vi "PrimaryInterfaceGetData.vi"(8 "PrimaryInterface":refnum<k24>, 11 "error in":errorcluster) -> (3 "error out":errorcluster)   [LabVIEW 2023, in "UnderAutomation.UniversalRobots.lvlib"]
uses:
  UnderAutomation.UniversalRobots.lvlib
  C:/Users/fg/Documents/UniversalRobots.vi/UnderAutomation.UniversalRobots/lib/UnderAutomation.UniversalRobots.dll
  lib/UnderAutomation.UniversalRobots.dll
panel:
  out "Data":T1
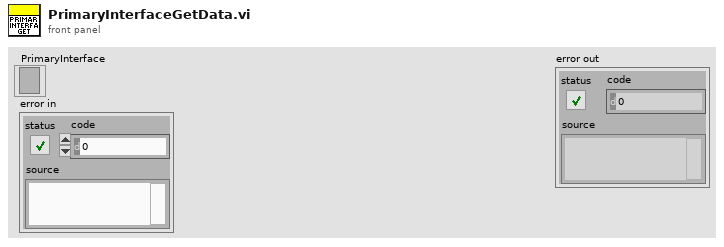
[diagram p1: front panel]
types:
  T1 = cluster{cluster{"FreedriveButtonEnabled":bool, "FreedriveButtonPressed":bool, "IOEnabledFreedrive":bool}, cluster{"Fx":dbl, "Fy":dbl, "Fz":dbl, "Frx":dbl, "Fry":dbl, "Frz":dbl}, cluster{"X":dbl, "Y":dbl, "Z":dbl, "Rx":dbl, "Ry":dbl, "Rz":dbl, "TCPOffsetX":dbl, "TCPOffsetY":dbl, "TCPOffsetZ":dbl, "TCPOffsetRX":dbl, "TCPOffsetRY":dbl, "TCPOffsetRZ":dbl}, cluster{"AJointDefault":dbl, "AToolDefault":dbl, "ControllerBoxType":i32, "EqRadius":dbl, "MasterboardVersion":i32, "RobotSubType":i32, "RobotType":i32, "VJointDefault":dbl, "VToolDefault":dbl, cluster{"DHa":dbl, "DHalpha":dbl, "DHd":dbl, "DHtheta":dbl, "JointMaxAcceleration":dbl, "JointMaxLimit":dbl, "JointMaxSpeed":dbl, "JointMinLimit":dbl}, cluster{"DHa":dbl, "DHalpha":dbl, "DHd":dbl, "DHtheta":dbl, "JointMaxAcceleration":dbl, "JointMaxLimit":dbl, "JointMaxSpeed":dbl, "JointMinLimit":dbl}, cluster{"DHa":dbl, "DHalpha":dbl, "DHd":dbl, "DHtheta":dbl, "JointMaxAcceleration":dbl, "JointMaxLimit":dbl, "JointMaxSpeed":dbl, "JointMinLimit":dbl}, cluster{"DHa":dbl, "DHalpha":dbl, "DHd":dbl, "DHtheta":dbl, "JointMaxAcceleration":dbl, "JointMaxLimit":dbl, "JointMaxSpeed":dbl, "JointMinLimit":dbl}, cluster{"DHa":dbl, "DHalpha":dbl, "DHd":dbl, "DHtheta":dbl, "JointMaxAcceleration":dbl, "JointMaxLimit":dbl, "JointMaxSpeed":dbl, "JointMinLimit":dbl}, cluster{"DHa":dbl, "DHalpha":dbl, "DHd":dbl, "DHtheta":dbl, "JointMaxAcceleration":dbl, "JointMaxLimit":dbl, "JointMaxSpeed":dbl, "JointMinLimit":dbl}}, cluster{"X":dbl, "Y":dbl, "Z":dbl, "Rx":dbl, "Ry":dbl, "Rz":dbl, "RobotDexterity":dbl}, cluster{cluster{"ActualSpeed":dbl, "Current":sgl, "JointMode":u8, "Position":dbl, "TargetPosition":dbl, "Temperature":sgl, "Voltage":sgl}, cluster{"ActualSpeed":dbl, "Current":sgl, "JointMode":u8, "Position":dbl, "TargetPosition":dbl, "Temperature":sgl, "Voltage":sgl}, cluster{"ActualSpeed":dbl, "Current":sgl, "JointMode":u8, "Position":dbl, "TargetPosition":dbl, "Temperature":sgl, "Voltage":sgl}, cluster{"ActualSpeed":dbl, "Current":sgl, "JointMode":u8, "Position":dbl, "TargetPosition":dbl, "Temperature":sgl, "Voltage":sgl}, cluster{"ActualSpeed":dbl, "Current":sgl, "JointMode":u8, "Position":dbl, "TargetPosition":dbl, "Temperature":sgl, "Voltage":sgl}, cluster{"ActualSpeed":dbl, "Current":sgl, "JointMode":u8, "Position":dbl, "TargetPosition":dbl, "Temperature":sgl, "Voltage":sgl}}, cluster{"KeyTextMessage":string, "RobotMessageArgument":i32, "RobotMessageCode":i32, "RobotMessageTitle":string}, cluster{cluster{"Checksum":i32, "DHa":dbl, "Dhalpha":dbl, "DHd":dbl, "DHtheta":dbl}, cluster{"Checksum":i32, "DHa":dbl, "Dhalpha":dbl, "DHd":dbl, "DHtheta":dbl}, cluster{"Checksum":i32, "DHa":dbl, "Dhalpha":dbl, "DHd":dbl, "DHtheta":dbl}, cluster{"Checksum":i32, "DHa":dbl, "Dhalpha":dbl, "DHd":dbl, "DHtheta":dbl}, cluster{"Checksum":i32, "DHa":dbl, "Dhalpha":dbl, "DHd":dbl, "DHtheta":dbl}, cluster{"Checksum":i32, "DHa":dbl, "Dhalpha":dbl, "DHd":dbl, "DHtheta":dbl}, "CalibrationStatus":i32}, cluster{"AnalogInput0":dbl, "AnalogInput1":dbl, "AnalogInputRange0":i32, "AnalogInputRange1":i32, "AnalogOutput0":dbl, "AnalogOutput1":dbl, "AnalogOutputDomain0":i32, "AnalogOutputDomain1":i32, cluster{"Configurable0":bool, "Configurable1":bool, "Configurable2":bool, "Configurable3":bool, "Configurable4":bool, "Configurable5":bool, "Configurable6":bool, "Configurable7":bool, "Digital0":bool, "Digital1":bool, "Digital2":bool, "Digital3":bool, "Digital4":bool, "Digital5":bool, "Digital6":bool, "Digital7":bool, "ToolDigital0":bool, "ToolDigital1":bool, "Value":i32}, cluster{"Configurable0":bool, "Configurable1":bool, "Configurable2":bool, "Configurable3":bool, "Configurable4":bool, "Configurable5":bool, "Configurable6":bool, "Configurable7":bool, "Digital0":bool, "Digital1":bool, "Digital2":bool, "Digital3":bool, "Digital4":bool, "Digital5":bool, "Digital6":bool, "Digital7":bool, "ToolDigital0":bool, "ToolDigital1":bool, "Value":i32}, "Euromap67Installed":i8, "EuromapCurrent":sgl, "EuromapInputBits":i32, "EuromapOutputBits":i32, "EuromapVoltage":sgl, "InReducedMode":u8, "MasterboardTemperature":sgl, "MasterIOCurrent":sgl, "OperationalModeSelectorInput":u8, "RobotCurrent":sgl, "RobotVoltage48V":sgl, "Safetymode":u8, "ThreePositionEnablingDeviceInput":u8}, cluster{"Blocking":bool, "Error":bool, "PopupMessageTitle":string, "PopupTextMessage":string, "RequestedType":i32, "RequestId":u32, "Warning":bool}, cluster{"ControlMode":i32, "EmergencyStopped":bool, "PhysicalRobotConnected":bool, "ProgramPaused":bool, "ProgramRunning":bool, "ProtectiveStopped":bool, "RealRobotEnabled":bool, "RobotMode":i32, "RobotPowerOn":bool, "SpeedScaling":dbl, "TargetSpeedFraction":dbl, "TargetSpeedFractionLimit":dbl, "TotalMilliseconds":dbl}, cluster{"RuntimeExceptionTextMessage":string, "ScriptColumnNumber":i32, "ScriptLineNumber":i32}, cluster{"SingularitySeverity":u8, "SingularityType":u8}, cluster{"TextMessage":string}, cluster{"BaudRate":i32, "Parity":i32, "RxIdleChars":sgl, "TxIdleChars":sgl, "ToolCommunicationIsEnabled":bool, "StopBits":i32}, cluster{"AnalogInput2":dbl, "AnalogInput3":dbl, "AnalogInputRange2":i32, "AnalogInputRange3":i32, "ToolCurrent":sgl, "ToolMode":u8, "ToolOutputVoltage":i8, "ToolTemperature":sgl, "ToolVoltage48V":sgl}, cluster{"DigitalOutputMode0":i32, "DigitalOutputMode1":i32, "OutputMode":i32}, cluster{"MajorVersion":u8, "MinorVersion":u8, "BugfixVersion":i32, "BuildNumber":i32, "BuildDate":string, "ProjectName":string}}
  T2 = cluster{"X":dbl, "Y":dbl, "Z":dbl, "Rx":dbl, "Ry":dbl, "Rz":dbl, "TCPOffsetX":dbl, "TCPOffsetY":dbl, "TCPOffsetZ":dbl, "TCPOffsetRX":dbl, "TCPOffsetRY":dbl, "TCPOffsetRZ":dbl}
  T3 = cluster{"Blocking":bool, "Error":bool, "PopupMessageTitle":string, "PopupTextMessage":string, "RequestedType":i32, "RequestId":u32, "Warning":bool}
  T4 = cluster{"AnalogInput2":dbl, "AnalogInput3":dbl, "AnalogInputRange2":i32, "AnalogInputRange3":i32, "ToolCurrent":sgl, "ToolMode":u8, "ToolOutputVoltage":i8, "ToolTemperature":sgl, "ToolVoltage48V":sgl}
  T5 = cluster{"MajorVersion":u8, "MinorVersion":u8, "BugfixVersion":i32, "BuildNumber":i32, "BuildDate":string, "ProjectName":string}
  T6 = cluster{"X":dbl, "Y":dbl, "Z":dbl, "Rx":dbl, "Ry":dbl, "Rz":dbl, "RobotDexterity":dbl}
  T7 = cluster{"Fx":dbl, "Fy":dbl, "Fz":dbl, "Frx":dbl, "Fry":dbl, "Frz":dbl}
  T8 = cluster{"KeyTextMessage":string, "RobotMessageArgument":i32, "RobotMessageCode":i32, "RobotMessageTitle":string}
  T9 = cluster{"BaudRate":i32, "Parity":i32, "RxIdleChars":sgl, "TxIdleChars":sgl, "ToolCommunicationIsEnabled":bool, "StopBits":i32}
  T10 = cluster{"Configurable0":bool, "Configurable1":bool, "Configurable2":bool, "Configurable3":bool, "Configurable4":bool, "Configurable5":bool, "Configurable6":bool, "Configurable7":bool, "Digital0":bool, "Digital1":bool, "Digital2":bool, "Digital3":bool, "Digital4":bool, "Digital5":bool, "Digital6":bool, "Digital7":bool, "ToolDigital0":bool, "ToolDigital1":bool, "Value":i32}
  T11 = cluster{"ControlMode":i32, "EmergencyStopped":bool, "PhysicalRobotConnected":bool, "ProgramPaused":bool, "ProgramRunning":bool, "ProtectiveStopped":bool, "RealRobotEnabled":bool, "RobotMode":i32, "RobotPowerOn":bool, "SpeedScaling":dbl, "TargetSpeedFraction":dbl, "TargetSpeedFractionLimit":dbl, "TotalMilliseconds":dbl}
  T12 = cluster{"DHa":dbl, "DHalpha":dbl, "DHd":dbl, "DHtheta":dbl, "JointMaxAcceleration":dbl, "JointMaxLimit":dbl, "JointMaxSpeed":dbl, "JointMinLimit":dbl}
  T13 = cluster{"ActualSpeed":dbl, "Current":sgl, "JointMode":u8, "Position":dbl, "TargetPosition":dbl, "Temperature":sgl, "Voltage":sgl}
  T14 = cluster{"AJointDefault":dbl, "AToolDefault":dbl, "ControllerBoxType":i32, "EqRadius":dbl, "MasterboardVersion":i32, "RobotSubType":i32, "RobotType":i32, "VJointDefault":dbl, "VToolDefault":dbl, cluster{"DHa":dbl, "DHalpha":dbl, "DHd":dbl, "DHtheta":dbl, "JointMaxAcceleration":dbl, "JointMaxLimit":dbl, "JointMaxSpeed":dbl, "JointMinLimit":dbl}, cluster{"DHa":dbl, "DHalpha":dbl, "DHd":dbl, "DHtheta":dbl, "JointMaxAcceleration":dbl, "JointMaxLimit":dbl, "JointMaxSpeed":dbl, "JointMinLimit":dbl}, cluster{"DHa":dbl, "DHalpha":dbl, "DHd":dbl, "DHtheta":dbl, "JointMaxAcceleration":dbl, "JointMaxLimit":dbl, "JointMaxSpeed":dbl, "JointMinLimit":dbl}, cluster{"DHa":dbl, "DHalpha":dbl, "DHd":dbl, "DHtheta":dbl, "JointMaxAcceleration":dbl, "JointMaxLimit":dbl, "JointMaxSpeed":dbl, "JointMinLimit":dbl}, cluster{"DHa":dbl, "DHalpha":dbl, "DHd":dbl, "DHtheta":dbl, "JointMaxAcceleration":dbl, "JointMaxLimit":dbl, "JointMaxSpeed":dbl, "JointMinLimit":dbl}, cluster{"DHa":dbl, "DHalpha":dbl, "DHd":dbl, "DHtheta":dbl, "JointMaxAcceleration":dbl, "JointMaxLimit":dbl, "JointMaxSpeed":dbl, "JointMinLimit":dbl}}
  T15 = cluster{cluster{"ActualSpeed":dbl, "Current":sgl, "JointMode":u8, "Position":dbl, "TargetPosition":dbl, "Temperature":sgl, "Voltage":sgl}, cluster{"ActualSpeed":dbl, "Current":sgl, "JointMode":u8, "Position":dbl, "TargetPosition":dbl, "Temperature":sgl, "Voltage":sgl}, cluster{"ActualSpeed":dbl, "Current":sgl, "JointMode":u8, "Position":dbl, "TargetPosition":dbl, "Temperature":sgl, "Voltage":sgl}, cluster{"ActualSpeed":dbl, "Current":sgl, "JointMode":u8, "Position":dbl, "TargetPosition":dbl, "Temperature":sgl, "Voltage":sgl}, cluster{"ActualSpeed":dbl, "Current":sgl, "JointMode":u8, "Position":dbl, "TargetPosition":dbl, "Temperature":sgl, "Voltage":sgl}, cluster{"ActualSpeed":dbl, "Current":sgl, "JointMode":u8, "Position":dbl, "TargetPosition":dbl, "Temperature":sgl, "Voltage":sgl}}
  T16 = cluster{"Checksum":i32, "DHa":dbl, "Dhalpha":dbl, "DHd":dbl, "DHtheta":dbl}
  T17 = cluster{"AnalogInput0":dbl, "AnalogInput1":dbl, "AnalogInputRange0":i32, "AnalogInputRange1":i32, "AnalogOutput0":dbl, "AnalogOutput1":dbl, "AnalogOutputDomain0":i32, "AnalogOutputDomain1":i32, cluster{"Configurable0":bool, "Configurable1":bool, "Configurable2":bool, "Configurable3":bool, "Configurable4":bool, "Configurable5":bool, "Configurable6":bool, "Configurable7":bool, "Digital0":bool, "Digital1":bool, "Digital2":bool, "Digital3":bool, "Digital4":bool, "Digital5":bool, "Digital6":bool, "Digital7":bool, "ToolDigital0":bool, "ToolDigital1":bool, "Value":i32}, cluster{"Configurable0":bool, "Configurable1":bool, "Configurable2":bool, "Configurable3":bool, "Configurable4":bool, "Configurable5":bool, "Configurable6":bool, "Configurable7":bool, "Digital0":bool, "Digital1":bool, "Digital2":bool, "Digital3":bool, "Digital4":bool, "Digital5":bool, "Digital6":bool, "Digital7":bool, "ToolDigital0":bool, "ToolDigital1":bool, "Value":i32}, "Euromap67Installed":i8, "EuromapCurrent":sgl, "EuromapInputBits":i32, "EuromapOutputBits":i32, "EuromapVoltage":sgl, "InReducedMode":u8, "MasterboardTemperature":sgl, "MasterIOCurrent":sgl, "OperationalModeSelectorInput":u8, "RobotCurrent":sgl, "RobotVoltage48V":sgl, "Safetymode":u8, "ThreePositionEnablingDeviceInput":u8}
  T18 = cluster{"FreedriveButtonEnabled":bool, "FreedriveButtonPressed":bool, "IOEnabledFreedrive":bool}
  T19 = cluster{cluster{"Checksum":i32, "DHa":dbl, "Dhalpha":dbl, "DHd":dbl, "DHtheta":dbl}, cluster{"Checksum":i32, "DHa":dbl, "Dhalpha":dbl, "DHd":dbl, "DHtheta":dbl}, cluster{"Checksum":i32, "DHa":dbl, "Dhalpha":dbl, "DHd":dbl, "DHtheta":dbl}, cluster{"Checksum":i32, "DHa":dbl, "Dhalpha":dbl, "DHd":dbl, "DHtheta":dbl}, cluster{"Checksum":i32, "DHa":dbl, "Dhalpha":dbl, "DHd":dbl, "DHtheta":dbl}, cluster{"Checksum":i32, "DHa":dbl, "Dhalpha":dbl, "DHd":dbl, "DHtheta":dbl}, "CalibrationStatus":i32}
  T20 = cluster{"RuntimeExceptionTextMessage":string, "ScriptColumnNumber":i32, "ScriptLineNumber":i32}
  T21 = cluster{"SingularitySeverity":u8, "SingularityType":u8}
  T22 = cluster{"DigitalOutputMode0":i32, "DigitalOutputMode1":i32, "OutputMode":i32}
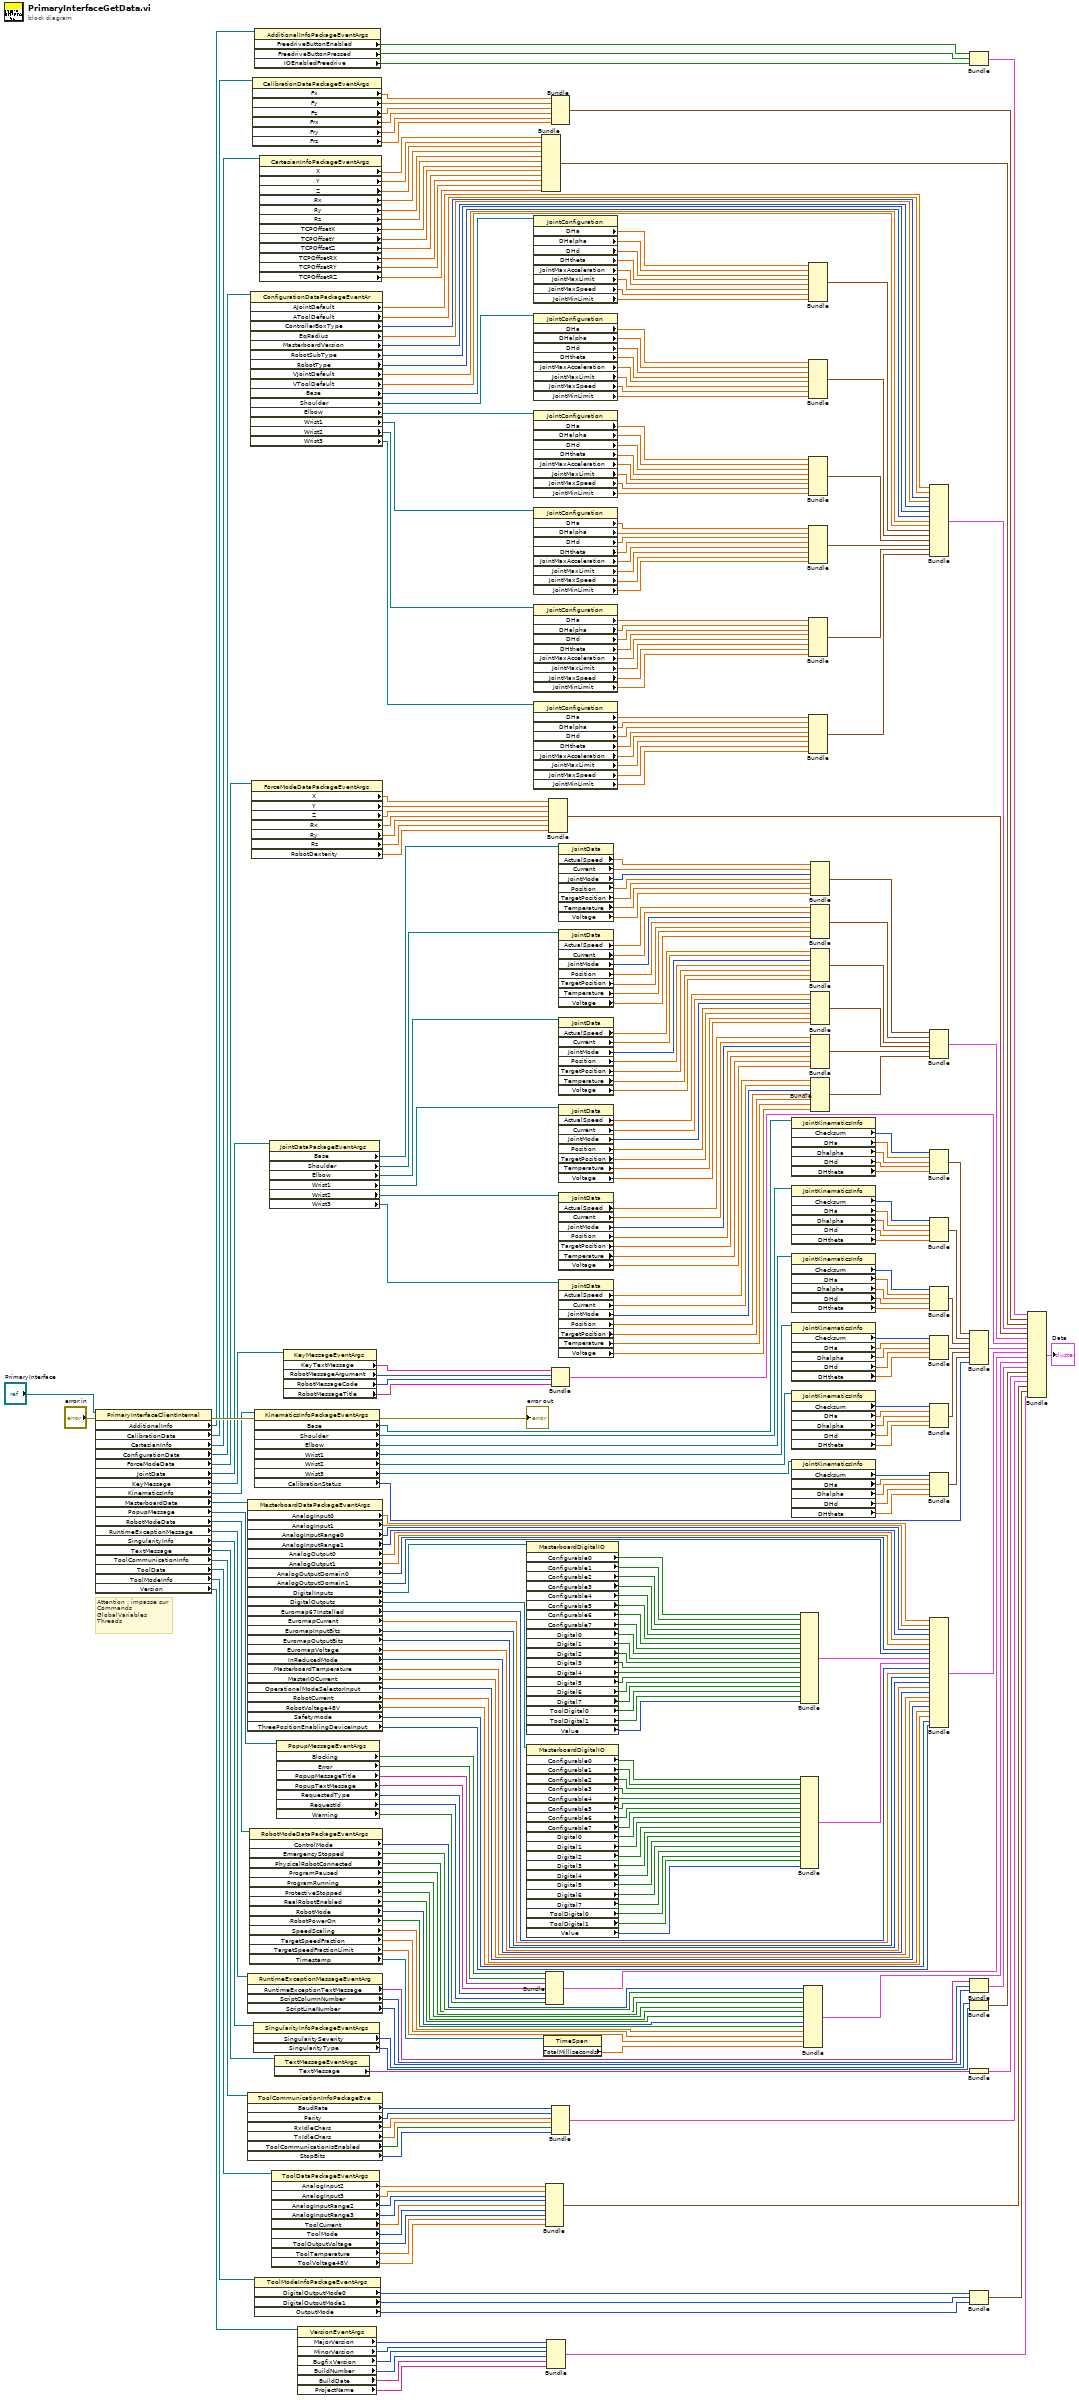
[diagram p0: block diagram]
diagram:
  # "Attention : impasse sur \nCommands\nGlobalVariables\nThreads"
  n1 = property class="PrimaryInterfaceClientInternal"(reference="PrimaryInterface", error in="error in") -> (error out=w233:errorcluster, "AdditionalInfo"=w206:refnum<k24>, "CalibrationData"=w203:refnum<k24>, "CartesianInfo"=w204:refnum<k24>, "ConfigurationData"=w208:refnum<k24>, "ForceModeData"=w205:refnum<k24>, "JointData"=w196:refnum<k24>, "KeyMessage"=w141:refnum<k24>, "KinematicsInfo"=w209:refnum<k24>, "MasterboardData"=w135:refnum<k24>, "PopupMessage"=w71:refnum<k24>, "RobotModeData"=w63:refnum<k24>, "RuntimeExceptionMessage"=w47:refnum<k24>, "SingularityInfo"=w43:refnum<k24>, "TextMessage"=w39:refnum<k24>, "ToolCommunicationInfo"=w36:refnum<k24>, "ToolData"=w28:refnum<k24>, "ToolModeInfo"=w18:refnum<k24>, "Version"=w207:refnum<k24>)  [unwired: 1 out]
  n2 = property class="MasterboardDataPackageEventArgs"(reference=w135) -> ("AnalogInput0"=w95:dbl, "AnalogInput1"=w94:dbl, "AnalogInputRange0"=w93:i32, "AnalogInputRange1"=w92:i32, "AnalogOutput0"=w91:dbl, "AnalogOutput1"=w90:dbl, "AnalogOutputDomain0"=w89:i32, "AnalogOutputDomain1"=w88:i32, "DigitalInputs"=w136:refnum<k24>, "DigitalOutputs"=w96:refnum<k24>, "Euromap67Installed"=w85:i8, "EuromapCurrent"=w84:sgl, "EuromapInputBits"=w83:i32, "EuromapOutputBits"=w82:i32, "EuromapVoltage"=w81:sgl, "InReducedMode"=w80:u8, "MasterboardTemperature"=w79:sgl, "MasterIOCurrent"=w78:sgl, "OperationalModeSelectorInput"=w77:u8, "RobotCurrent"=w76:sgl, "RobotVoltage48V"=w75:sgl, "Safetymode"=w74:u8, "ThreePositionEnablingDeviceInput"=w73:u8)  [unwired: 1 in, 2 out]
  n3 = property class="RuntimeExceptionMessageEventArg"(reference=w47) -> ("RuntimeExceptionTextMessage"=w50:string, "ScriptColumnNumber"=w49:i32, "ScriptLineNumber"=w48:i32)  [unwired: 1 in, 2 out]
  n4 = property class="ToolCommunicationInfoPackageEve"(reference=w36) -> ("BaudRate"=w35:i32, "Parity"=w34:i32, "RxIdleChars"=w33:sgl, "TxIdleChars"=w32:sgl, "ToolCommunicationIsEnabled"=w31:bool, "StopBits"=w30:i32)  [unwired: 1 in, 2 out]
  n5 = property class="RobotModeDataPackageEventArgs"(reference=w63) -> ("ControlMode"=w62:i32, "EmergencyStopped"=w61:bool, "PhysicalRobotConnected"=w60:bool, "ProgramPaused"=w59:bool, "ProgramRunning"=w58:bool, "ProtectiveStopped"=w57:bool, "RealRobotEnabled"=w56:bool, "RobotMode"=w55:i32, "RobotPowerOn"=w54:bool, "SpeedScaling"=w53:dbl, "TargetSpeedFraction"=w52:dbl, "TargetSpeedFractionLimit"=w51:dbl, "Timestamp"=w10:refnum<k24>)  [unwired: 1 in, 2 out]
  n6 = property class="ConfigurationDataPackageEventAr"(reference=w208) -> ("AJointDefault"=w298:dbl, "AToolDefault"=w297:dbl, "ControllerBoxType"=w296:i32, "EqRadius"=w295:dbl, "MasterboardVersion"=w294:i32, "RobotSubType"=w293:i32, "RobotType"=w292:i32, "VJointDefault"=w291:dbl, "VToolDefault"=w290:dbl, "Base"=w352:refnum<k24>, "Shoulder"=w303:refnum<k24>, "Elbow"=w302:refnum<k24>, "Wrist1"=w301:refnum<k24>, "Wrist2"=w300:refnum<k24>, "Wrist3"=w299:refnum<k24>)  [unwired: 1 in, 2 out]
  n7 = property class="ForceModeDataPackageEventArgs"(reference=w205) -> ("X"=w216:dbl, "Y"=w215:dbl, "Z"=w214:dbl, "Rx"=w213:dbl, "Ry"=w212:dbl, "Rz"=w211:dbl, "RobotDexterity"=w210:dbl)  [unwired: 1 in, 2 out]
  n8 = property class="CalibrationDataPackageEventArgs"(reference=w203) -> ("Fx"=w202:dbl, "Fy"=w201:dbl, "Fz"=w200:dbl, "Frx"=w199:dbl, "Fry"=w198:dbl, "Frz"=w197:dbl)  [unwired: 1 in, 2 out]
  n9 = property class="SingularityInfoPackageEventArgs"(reference=w43) -> ("SingularitySeverity"=w42:u8, "SingularityType"=w41:u8)  [unwired: 1 in, 2 out]
  n10 = property class="KinematicsInfoPackageEventArgs"(reference=w209, error in=w233) -> (error out=→"error out":errorcluster, "Base"=w283:refnum<k24>, "Shoulder"=w252:refnum<k24>, "Elbow"=w251:refnum<k24>, "Wrist1"=w250:refnum<k24>, "Wrist2"=w249:refnum<k24>, "Wrist3"=w248:refnum<k24>, "CalibrationStatus"=w241:i32)  [unwired: 1 out]
  n11 = property class="AdditionalInfoPackageEventArgs"(reference=w206) -> ("FreedriveButtonEnabled"=w231:bool, "FreedriveButtonPressed"=w230:bool, "IOEnabledFreedrive"=w229:bool)  [unwired: 1 in, 2 out]
  n12 = property class="ToolModeInfoPackageEventArgs"(reference=w18) -> ("DigitalOutputMode0"=w17:i32, "DigitalOutputMode1"=w16:i32, "OutputMode"=w15:i32)  [unwired: 1 in, 2 out]
  n13 = property class="CartesianInfoPackageEventArgs"(reference=w204) -> ("X"=w228:dbl, "Y"=w227:dbl, "Z"=w226:dbl, "Rx"=w225:dbl, "Ry"=w224:dbl, "Rz"=w223:dbl, "TCPOffsetX"=w222:dbl, "TCPOffsetY"=w220:dbl, "TCPOffsetZ"=w221:dbl, "TCPOffsetRX"=w218:dbl, "TCPOffsetRY"=w219:dbl, "TCPOffsetRZ"=w217:dbl)  [unwired: 1 in, 2 out]
  n14 = property class="JointDataPackageEventArgs"(reference=w196) -> ("Base"=w195:refnum<k24>, "Shoulder"=w152:refnum<k24>, "Elbow"=w151:refnum<k24>, "Wrist1"=w150:refnum<k24>, "Wrist2"=w149:refnum<k24>, "Wrist3"=w148:refnum<k24>)  [unwired: 1 in, 2 out]
  n15 = property class="ToolDataPackageEventArgs"(reference=w28) -> ("AnalogInput2"=w27:dbl, "AnalogInput3"=w26:dbl, "AnalogInputRange2"=w25:i32, "AnalogInputRange3"=w24:i32, "ToolCurrent"=w23:sgl, "ToolMode"=w22:u8, "ToolOutputVoltage"=w21:i8, "ToolTemperature"=w20:sgl, "ToolVoltage48V"=w19:sgl)  [unwired: 1 in, 2 out]
  n16 = property class="TextMessageEventArgs"(reference=w39) -> ("TextMessage"=w38:string)  [unwired: 1 in, 2 out]
  n17 = property class="PopupMessageEventArgs"(reference=w71) -> ("Blocking"=w70:bool, "Error"=w69:bool, "PopupMessageTitle"=w68:string, "PopupTextMessage"=w67:string, "RequestedType"=w66:i32, "RequestId"=w65:u32, "Warning"=w64:bool)  [unwired: 1 in, 2 out]
  n18 = property class="KeyMessageEventArgs"(reference=w141) -> ("KeyTextMessage"=w140:string, "RobotMessageArgument"=w139:i32, "RobotMessageCode"=w138:i32, "RobotMessageTitle"=w137:string)  [unwired: 1 in, 2 out]
  n19 = property class="VersionEventArgs"(reference=w207) -> ("MajorVersion"=w240:u8, "MinorVersion"=w239:u8, "BugfixVersion"=w238:i32, "BuildNumber"=w237:i32, "BuildDate"=w236:string, "ProjectName"=w235:string)  [unwired: 1 in, 2 out]
  n20 = property class="MasterboardDigitalIO"(reference=w136) -> ("Configurable0"=w134:bool, "Configurable1"=w133:bool, "Configurable2"=w132:bool, "Configurable3"=w131:bool, "Configurable4"=w130:bool, "Configurable5"=w129:bool, "Configurable6"=w128:bool, "Configurable7"=w127:bool, "Digital0"=w126:bool, "Digital1"=w125:bool, "Digital2"=w124:bool, "Digital3"=w123:bool, "Digital4"=w122:bool, "Digital5"=w121:bool, "Digital6"=w120:bool, "Digital7"=w119:bool, "ToolDigital0"=w118:bool, "ToolDigital1"=w117:bool, "Value"=w116:i32)  [unwired: 1 in, 2 out]
  n21 = property class="MasterboardDigitalIO"(reference=w96) -> ("Configurable0"=w97:bool, "Configurable1"=w98:bool, "Configurable2"=w99:bool, "Configurable3"=w100:bool, "Configurable4"=w101:bool, "Configurable5"=w102:bool, "Configurable6"=w103:bool, "Configurable7"=w104:bool, "Digital0"=w105:bool, "Digital1"=w106:bool, "Digital2"=w107:bool, "Digital3"=w108:bool, "Digital4"=w109:bool, "Digital5"=w110:bool, "Digital6"=w111:bool, "Digital7"=w112:bool, "ToolDigital0"=w113:bool, "ToolDigital1"=w114:bool, "Value"=w115:i32)  [unwired: 1 in, 2 out]
  n22 = property class="JointConfiguration"(reference=w352) -> ("DHa"=w351:dbl, "DHalpha"=w350:dbl, "DHd"=w349:dbl, "DHtheta"=w347:dbl, "JointMaxAcceleration"=w348:dbl, "JointMaxLimit"=w346:dbl, "JointMaxSpeed"=w345:dbl, "JointMinLimit"=w344:dbl)  [unwired: 1 in, 2 out]
  n23 = property class="JointConfiguration"(reference=w303) -> ("DHa"=w304:dbl, "DHalpha"=w305:dbl, "DHd"=w306:dbl, "DHtheta"=w308:dbl, "JointMaxAcceleration"=w307:dbl, "JointMaxLimit"=w309:dbl, "JointMaxSpeed"=w310:dbl, "JointMinLimit"=w311:dbl)  [unwired: 1 in, 2 out]
  n24 = property class="JointConfiguration"(reference=w302) -> ("DHa"=w319:dbl, "DHalpha"=w318:dbl, "DHd"=w317:dbl, "DHtheta"=w315:dbl, "JointMaxAcceleration"=w316:dbl, "JointMaxLimit"=w314:dbl, "JointMaxSpeed"=w313:dbl, "JointMinLimit"=w312:dbl)  [unwired: 1 in, 2 out]
  n25 = property class="JointConfiguration"(reference=w301) -> ("DHa"=w336:dbl, "DHalpha"=w337:dbl, "DHd"=w338:dbl, "DHtheta"=w340:dbl, "JointMaxAcceleration"=w339:dbl, "JointMaxLimit"=w341:dbl, "JointMaxSpeed"=w342:dbl, "JointMinLimit"=w343:dbl)  [unwired: 1 in, 2 out]
  n26 = property class="JointConfiguration"(reference=w300) -> ("DHa"=w335:dbl, "DHalpha"=w334:dbl, "DHd"=w333:dbl, "DHtheta"=w331:dbl, "JointMaxAcceleration"=w332:dbl, "JointMaxLimit"=w330:dbl, "JointMaxSpeed"=w329:dbl, "JointMinLimit"=w328:dbl)  [unwired: 1 in, 2 out]
  n27 = property class="JointConfiguration"(reference=w299) -> ("DHa"=w320:dbl, "DHalpha"=w321:dbl, "DHd"=w322:dbl, "DHtheta"=w324:dbl, "JointMaxAcceleration"=w323:dbl, "JointMaxLimit"=w325:dbl, "JointMaxSpeed"=w326:dbl, "JointMinLimit"=w327:dbl)  [unwired: 1 in, 2 out]
  n28 = Bundle("X"=w228, "Y"=w227, "Z"=w226, "Rx"=w225, "Ry"=w224, "Rz"=w223, "TCPOffsetX"=w222, "TCPOffsetY"=w220, "TCPOffsetZ"=w221, "TCPOffsetRX"=w218, "TCPOffsetRY"=w219, "TCPOffsetRZ"=w217) -> (w5:T2)  [unwired: 1 in]
  n29 = property class="TimeSpan"(reference=w10) -> ("TotalMilliseconds"=w11:dbl)  [unwired: 1 in, 2 out]
  n30 = Bundle("Blocking"=w70, "Error"=w69, "PopupMessageTitle"=w68, "PopupTextMessage"=w67, "RequestedType"=w66, "RequestId"=w65, "Warning"=w64) -> (w46:T3)  [unwired: 1 in]
  n31 = Bundle("AnalogInput2"=w27, "AnalogInput3"=w26, "AnalogInputRange2"=w25, "AnalogInputRange3"=w24, "ToolCurrent"=w23, "ToolMode"=w22, "ToolOutputVoltage"=w21, "ToolTemperature"=w20, "ToolVoltage48V"=w19) -> (w14:T4)  [unwired: 1 in]
  n32 = Bundle("MajorVersion"=w240, "MinorVersion"=w239, "BugfixVersion"=w238, "BuildNumber"=w237, "BuildDate"=w236, "ProjectName"=w235) -> (w12:T5)  [unwired: 1 in]
  n33 = Bundle("X"=w216, "Y"=w215, "Z"=w214, "Rx"=w213, "Ry"=w212, "Rz"=w211, "RobotDexterity"=w210) -> (w7:T6)  [unwired: 1 in]
  n34 = Bundle("Fx"=w202, "Fy"=w201, "Fz"=w200, "Frx"=w199, "Fry"=w198, "Frz"=w197) -> (w4:T7)  [unwired: 1 in]
  n35 = Bundle("KeyTextMessage"=w140, "RobotMessageArgument"=w139, "RobotMessageCode"=w138, "RobotMessageTitle"=w137) -> (w9:T8)  [unwired: 1 in]
  n36 = Bundle("BaudRate"=w35, "Parity"=w34, "RxIdleChars"=w33, "TxIdleChars"=w32, "ToolCommunicationIsEnabled"=w31, "StopBits"=w30) -> (w29:T9)  [unwired: 1 in]
  n37 = property class="JointData"(reference=w195) -> ("ActualSpeed"=w194:dbl, "Current"=w193:sgl, "JointMode"=w192:u8, "Position"=w191:dbl, "TargetPosition"=w190:dbl, "Temperature"=w189:sgl, "Voltage"=w188:sgl)  [unwired: 1 in, 2 out]
  n38 = property class="JointData"(reference=w152) -> ("ActualSpeed"=w181:dbl, "Current"=w182:sgl, "JointMode"=w183:u8, "Position"=w184:dbl, "TargetPosition"=w185:dbl, "Temperature"=w186:sgl, "Voltage"=w187:sgl)  [unwired: 1 in, 2 out]
  n39 = property class="JointData"(reference=w151) -> ("ActualSpeed"=w180:dbl, "Current"=w179:sgl, "JointMode"=w178:u8, "Position"=w177:dbl, "TargetPosition"=w176:dbl, "Temperature"=w175:sgl, "Voltage"=w174:sgl)  [unwired: 1 in, 2 out]
  n40 = property class="JointData"(reference=w150) -> ("ActualSpeed"=w153:dbl, "Current"=w154:sgl, "JointMode"=w155:u8, "Position"=w156:dbl, "TargetPosition"=w157:dbl, "Temperature"=w158:sgl, "Voltage"=w159:sgl)  [unwired: 1 in, 2 out]
  n41 = property class="JointData"(reference=w149) -> ("ActualSpeed"=w166:dbl, "Current"=w165:sgl, "JointMode"=w164:u8, "Position"=w163:dbl, "TargetPosition"=w162:dbl, "Temperature"=w161:sgl, "Voltage"=w160:sgl)  [unwired: 1 in, 2 out]
  n42 = property class="JointData"(reference=w148) -> ("ActualSpeed"=w167:dbl, "Current"=w168:sgl, "JointMode"=w169:u8, "Position"=w170:dbl, "TargetPosition"=w171:dbl, "Temperature"=w172:sgl, "Voltage"=w173:sgl)  [unwired: 1 in, 2 out]
  n43 = property class="JointKinematicsInfo"(reference=w283) -> ("Checksum"=w282:i32, "DHa"=w281:dbl, "Dhalpha"=w280:dbl, "DHd"=w279:dbl, "DHtheta"=w278:dbl)  [unwired: 1 in, 2 out]
  n44 = property class="JointKinematicsInfo"(reference=w252) -> ("Checksum"=w273:i32, "DHa"=w274:dbl, "Dhalpha"=w275:dbl, "DHd"=w276:dbl, "DHtheta"=w277:dbl)  [unwired: 1 in, 2 out]
  n45 = property class="JointKinematicsInfo"(reference=w251) -> ("Checksum"=w272:i32, "DHa"=w271:dbl, "Dhalpha"=w270:dbl, "DHd"=w269:dbl, "DHtheta"=w268:dbl)  [unwired: 1 in, 2 out]
  n46 = property class="JointKinematicsInfo"(reference=w250) -> ("Checksum"=w263:i32, "DHa"=w264:dbl, "Dhalpha"=w265:dbl, "DHd"=w266:dbl, "DHtheta"=w267:dbl)  [unwired: 1 in, 2 out]
  n47 = property class="JointKinematicsInfo"(reference=w249) -> ("Checksum"=w262:i32, "DHa"=w261:dbl, "Dhalpha"=w260:dbl, "DHd"=w259:dbl, "DHtheta"=w258:dbl)  [unwired: 1 in, 2 out]
  n48 = property class="JointKinematicsInfo"(reference=w248) -> ("Checksum"=w253:i32, "DHa"=w254:dbl, "Dhalpha"=w255:dbl, "DHd"=w256:dbl, "DHtheta"=w257:dbl)  [unwired: 1 in, 2 out]
  n49 = Bundle("Configurable0"=w134, "Configurable1"=w133, "Configurable2"=w132, "Configurable3"=w131, "Configurable4"=w130, "Configurable5"=w129, "Configurable6"=w128, "Configurable7"=w127, "Digital0"=w126, "Digital1"=w125, "Digital2"=w124, "Digital3"=w123, "Digital4"=w122, "Digital5"=w121, "Digital6"=w120, "Digital7"=w119, "ToolDigital0"=w118, "ToolDigital1"=w117, "Value"=w116) -> (w87:T10)  [unwired: 1 in]
  n50 = Bundle("Configurable0"=w97, "Configurable1"=w98, "Configurable2"=w99, "Configurable3"=w100, "Configurable4"=w101, "Configurable5"=w102, "Configurable6"=w103, "Configurable7"=w104, "Digital0"=w105, "Digital1"=w106, "Digital2"=w107, "Digital3"=w108, "Digital4"=w109, "Digital5"=w110, "Digital6"=w111, "Digital7"=w112, "ToolDigital0"=w113, "ToolDigital1"=w114, "Value"=w115) -> (w86:T10)  [unwired: 1 in]
  n51 = Bundle("ControlMode"=w62, "EmergencyStopped"=w61, "PhysicalRobotConnected"=w60, "ProgramPaused"=w59, "ProgramRunning"=w58, "ProtectiveStopped"=w57, "RealRobotEnabled"=w56, "RobotMode"=w55, "RobotPowerOn"=w54, "SpeedScaling"=w53, "TargetSpeedFraction"=w52, "TargetSpeedFractionLimit"=w51, "TotalMilliseconds"=w11) -> (w45:T11)  [unwired: 1 in]
  n52 = Bundle("DHa"=w351, "DHalpha"=w350, "DHd"=w349, "DHtheta"=w347, "JointMaxAcceleration"=w348, "JointMaxLimit"=w346, "JointMaxSpeed"=w345, "JointMinLimit"=w344) -> (w289:T12)  [unwired: 1 in]
  n53 = Bundle("DHa"=w304, "DHalpha"=w305, "DHd"=w306, "DHtheta"=w308, "JointMaxAcceleration"=w307, "JointMaxLimit"=w309, "JointMaxSpeed"=w310, "JointMinLimit"=w311) -> (w288:T12)  [unwired: 1 in]
  n54 = Bundle("DHa"=w319, "DHalpha"=w318, "DHd"=w317, "DHtheta"=w315, "JointMaxAcceleration"=w316, "JointMaxLimit"=w314, "JointMaxSpeed"=w313, "JointMinLimit"=w312) -> (w287:T12)  [unwired: 1 in]
  n55 = Bundle("DHa"=w336, "DHalpha"=w337, "DHd"=w338, "DHtheta"=w340, "JointMaxAcceleration"=w339, "JointMaxLimit"=w341, "JointMaxSpeed"=w342, "JointMinLimit"=w343) -> (w286:T12)  [unwired: 1 in]
  n56 = Bundle("DHa"=w335, "DHalpha"=w334, "DHd"=w333, "DHtheta"=w331, "JointMaxAcceleration"=w332, "JointMaxLimit"=w330, "JointMaxSpeed"=w329, "JointMinLimit"=w328) -> (w285:T12)  [unwired: 1 in]
  n57 = Bundle("DHa"=w320, "DHalpha"=w321, "DHd"=w322, "DHtheta"=w324, "JointMaxAcceleration"=w323, "JointMaxLimit"=w325, "JointMaxSpeed"=w326, "JointMinLimit"=w327) -> (w284:T12)  [unwired: 1 in]
  n58 = Bundle("ActualSpeed"=w194, "Current"=w193, "JointMode"=w192, "Position"=w191, "TargetPosition"=w190, "Temperature"=w189, "Voltage"=w188) -> (w147:T13)  [unwired: 1 in]
  n59 = Bundle("ActualSpeed"=w181, "Current"=w182, "JointMode"=w183, "Position"=w184, "TargetPosition"=w185, "Temperature"=w186, "Voltage"=w187) -> (w146:T13)  [unwired: 1 in]
  n60 = Bundle("ActualSpeed"=w180, "Current"=w179, "JointMode"=w178, "Position"=w177, "TargetPosition"=w176, "Temperature"=w175, "Voltage"=w174) -> (w145:T13)  [unwired: 1 in]
  n61 = Bundle("ActualSpeed"=w153, "Current"=w154, "JointMode"=w155, "Position"=w156, "TargetPosition"=w157, "Temperature"=w158, "Voltage"=w159) -> (w144:T13)  [unwired: 1 in]
  n62 = Bundle("ActualSpeed"=w166, "Current"=w165, "JointMode"=w164, "Position"=w163, "TargetPosition"=w162, "Temperature"=w161, "Voltage"=w160) -> (w143:T13)  [unwired: 1 in]
  n63 = Bundle("ActualSpeed"=w167, "Current"=w168, "JointMode"=w169, "Position"=w170, "TargetPosition"=w171, "Temperature"=w172, "Voltage"=w173) -> (w142:T13)  [unwired: 1 in]
  n64 = Bundle("AJointDefault"=w298, "AToolDefault"=w297, "ControllerBoxType"=w296, "EqRadius"=w295, "MasterboardVersion"=w294, "RobotSubType"=w293, "RobotType"=w292, "VJointDefault"=w291, "VToolDefault"=w290, w289, w288, w287, w286, w285, w284) -> (w6:T14)  [unwired: 1 in]
  n65 = Bundle(w147, w146, w145, w144, w143, w142) -> (w8:T15)  [unwired: 1 in]
  n66 = Bundle("Checksum"=w282, "DHa"=w281, "Dhalpha"=w280, "DHd"=w279, "DHtheta"=w278) -> (w247:T16)  [unwired: 1 in]
  n67 = Bundle("Checksum"=w273, "DHa"=w274, "Dhalpha"=w275, "DHd"=w276, "DHtheta"=w277) -> (w246:T16)  [unwired: 1 in]
  n68 = Bundle("Checksum"=w272, "DHa"=w271, "Dhalpha"=w270, "DHd"=w269, "DHtheta"=w268) -> (w245:T16)  [unwired: 1 in]
  n69 = Bundle("Checksum"=w263, "DHa"=w264, "Dhalpha"=w265, "DHd"=w266, "DHtheta"=w267) -> (w244:T16)  [unwired: 1 in]
  n70 = Bundle("Checksum"=w262, "DHa"=w261, "Dhalpha"=w260, "DHd"=w259, "DHtheta"=w258) -> (w243:T16)  [unwired: 1 in]
  n71 = Bundle("Checksum"=w253, "DHa"=w254, "Dhalpha"=w255, "DHd"=w256, "DHtheta"=w257) -> (w242:T16)  [unwired: 1 in]
  n72 = Bundle("AnalogInput0"=w95, "AnalogInput1"=w94, "AnalogInputRange0"=w93, "AnalogInputRange1"=w92, "AnalogOutput0"=w91, "AnalogOutput1"=w90, "AnalogOutputDomain0"=w89, "AnalogOutputDomain1"=w88, w87, w86, "Euromap67Installed"=w85, "EuromapCurrent"=w84, "EuromapInputBits"=w83, "EuromapOutputBits"=w82, "EuromapVoltage"=w81, "InReducedMode"=w80, "MasterboardTemperature"=w79, "MasterIOCurrent"=w78, "OperationalModeSelectorInput"=w77, "RobotCurrent"=w76, "RobotVoltage48V"=w75, "Safetymode"=w74, "ThreePositionEnablingDeviceInput"=w73) -> (w72:T17)  [unwired: 1 in]
  n73 = Bundle("FreedriveButtonEnabled"=w231, "FreedriveButtonPressed"=w230, "IOEnabledFreedrive"=w229) -> (w3:T18)  [unwired: 1 in]
  n74 = Bundle(w247, w246, w245, w244, w243, w242, "CalibrationStatus"=w241) -> (w2:T19)  [unwired: 1 in]
  n75 = Bundle("RuntimeExceptionTextMessage"=w50, "ScriptColumnNumber"=w49, "ScriptLineNumber"=w48) -> (w44:T20)  [unwired: 1 in]
  n76 = Bundle("SingularitySeverity"=w42, "SingularityType"=w41) -> (w40:T21)  [unwired: 1 in]
  n77 = Bundle("TextMessage"=w38) -> (w37:cluster{"TextMessage":string})  [unwired: 1 in]
  n78 = Bundle("DigitalOutputMode0"=w17, "DigitalOutputMode1"=w16, "OutputMode"=w15) -> (w13:T22)  [unwired: 1 in]
  n79 = Bundle(w3, w4, w5, w6, w7, w8, w9, w2, w72, w46, w45, w44, w40, w37, w29, w14, w13, w12) -> (→"Data":T1)  [unwired: 1 in]
